vi "Init Little.vi"() -> (2 "Little Boat Queues":T1)   [LabVIEW 2013]
uses:
  Data/TypeDefs/UTM Location.ctl
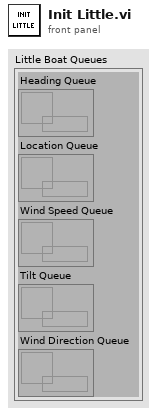
[diagram p1: front panel]
types:
  T1 = cluster{"Heading Queue":refnum<queue>, "Location Queue":refnum<queue>, "Wind Speed Queue":refnum<queue>, "Tilt Queue":refnum<queue>, "Wind Direction Queue":refnum<queue>}
  T2 = typedef "UTM Location.ctl" = cluster{"UTM Zone":dbl, "Hemisphere":enum16{"North", "South"}, "East":dbl, "North":dbl}
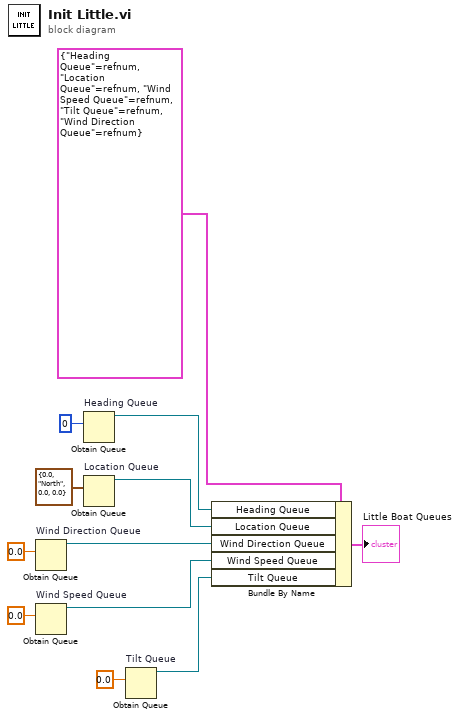
[diagram p0: block diagram]
diagram:
  n1 = Obtain Queue "Wind Direction Queue"(element data type=0.0) -> (queue out=w4:refnum<queue>)  [unwired: 4 in, 2 out]
  n2 = Obtain Queue "Wind Speed Queue"(element data type=0.0) -> (queue out=w3:refnum<queue>)  [unwired: 4 in, 2 out]
  n3 = Obtain Queue "Heading Queue"(element data type=0) -> (queue out=w11:refnum<queue>)  [unwired: 4 in, 2 out]
  n4 = Obtain Queue "Location Queue"(element data type=T2 {"UTM Zone"=0.0, "Hemisphere"=enum."North", "East"=0.0, "North"=0.0} ("UTM Location")) -> (queue out=w5:refnum<queue>)  [unwired: 4 in, 2 out]
  n5 = Obtain Queue "Tilt Queue"(element data type=0.0) -> (queue out=w2:refnum<queue>)  [unwired: 4 in, 2 out]
  n6 = Bundle By Name(cluster=T1 {"Heading Queue"=refnum, "Location Queue"=refnum, "Wind Speed Queue"=refnum, "Tilt Queue"=refnum, "Wind Direction Queue"=refnum} ("input cluster"), "Heading Queue"=w11, "Location Queue"=w5, "Wind Direction Queue"=w4, "Wind Speed Queue"=w3, "Tilt Queue"=w2) -> (→"Little Boat Queues":T1)
